vi "BlackBox232.vi"(5 "Input Command":string, 6 "VISA resource name":refnum<visa-resource-name>) -> (0 "error out 3":errorcluster, 1 "MonData":T2, 2 "MeasData":T1, 3 "Boolean":bool, 4 "String":string)   [LabVIEW 2010]
uses:
  <vilib>/Instr/_visa.llb/VISA Configure Serial Port (Instr).vi
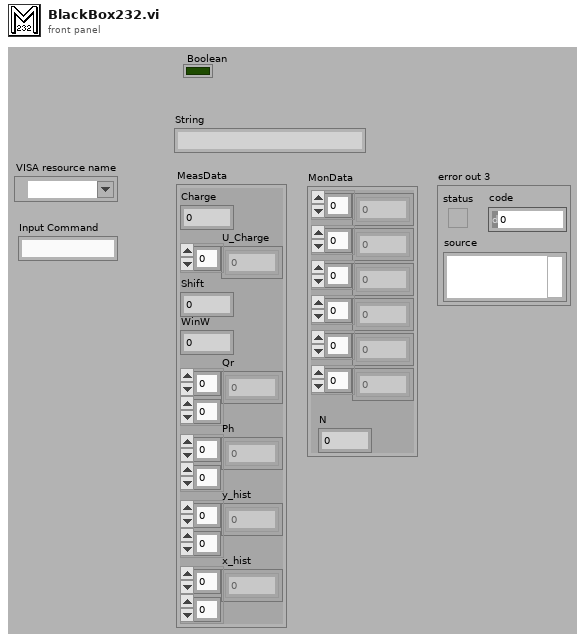
[diagram p1: front panel]
types:
  T1 = cluster{"Charge":i32, "U_Charge":i32[], "Shift":i32, "WinW":i32, "Qr":i32[][], "Ph":i32[][], "y_hist":i32[][], "x_hist":i32[][]}
  T2 = cluster{u16[], u16[], u16[], u16[], u16[], u16[], "N":i32}
  T3 = cluster{"Charge":i32, " U_Charge ":i32[], "Shift":i32, "WinW":i32, "Qr":i32[][], "Ph":i32[][], "y_hist":i32[][], "x_hist":i32[][]}
  T4 = cluster{u16[], u16[], u16[], u16[], u16[], u16[], dbl}
  T5 = cluster{u16[], u16[], u16[], u16[], u16[], u16[], "N":dbl}
  T6 = cluster{u16[], u16[], u16[], u16[], u16[], u16[], "Numeric":dbl}
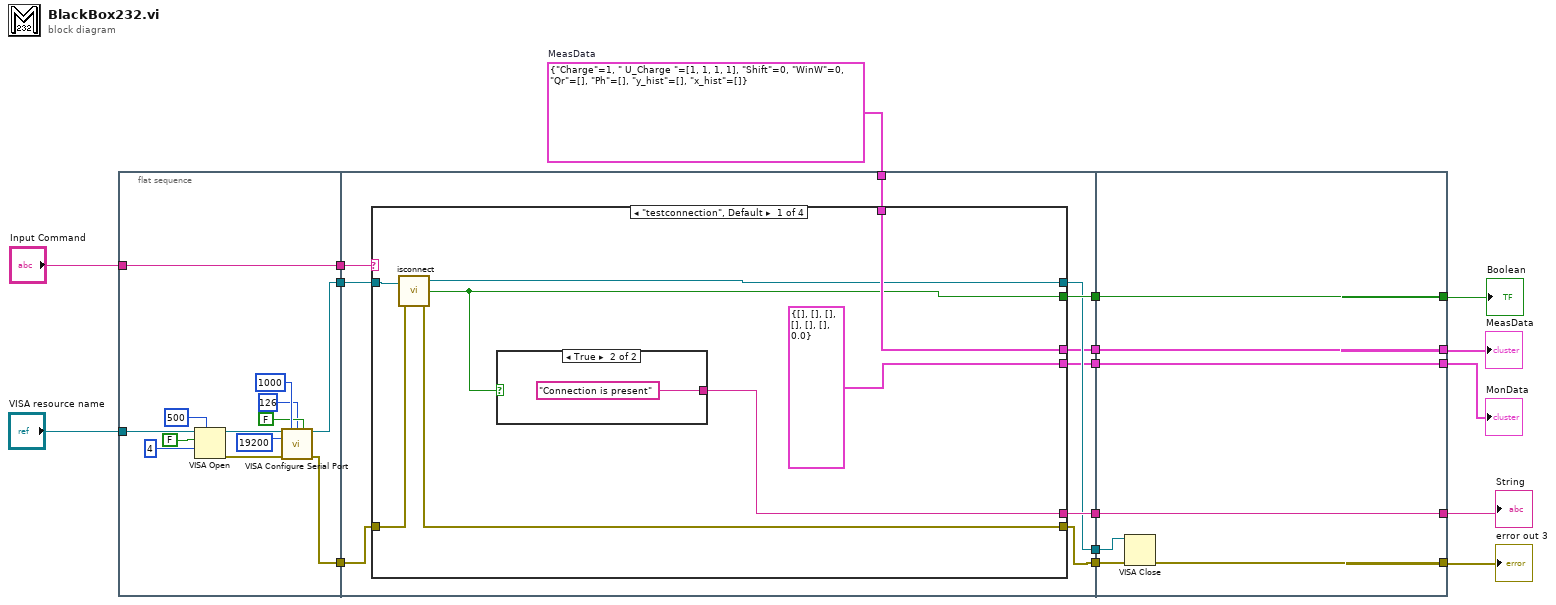
[diagram p0: block diagram]
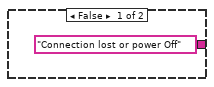
[diagram p2: hidden frame]
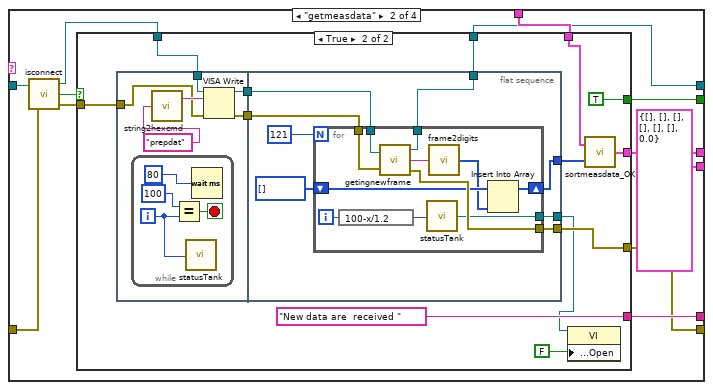
[diagram p3: hidden frame]
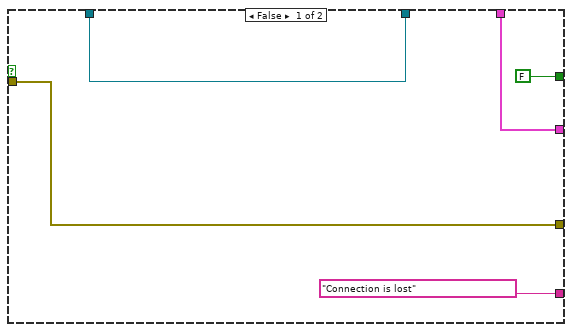
[diagram p4: hidden frame]
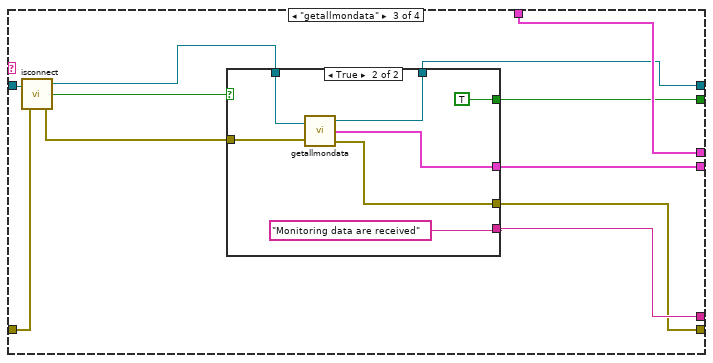
[diagram p5: hidden frame]
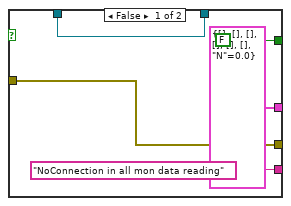
[diagram p6: hidden frame]
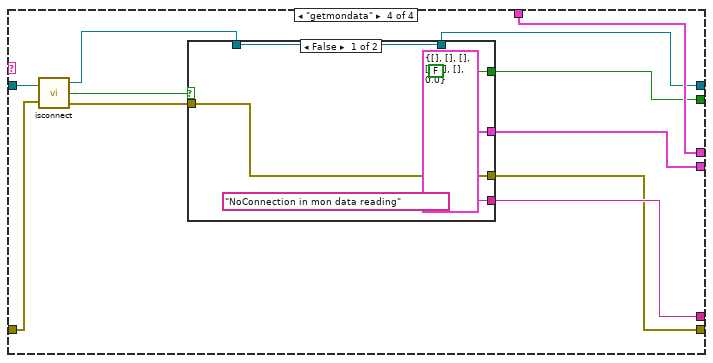
[diagram p7: hidden frame]
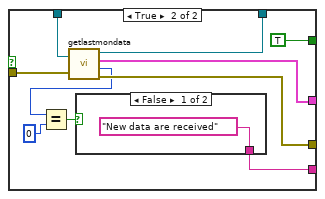
[diagram p8: hidden frame]
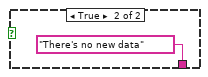
[diagram p9: hidden frame]
diagram:
  w3 = T3 {"Charge"=1, " U_Charge "=[1, 1, 1, 1], "Shift"=0, "WinW"=0, "Qr"=[], "Ph"=[], "y_hist"=[], "x_hist"=[]}  # MeasData
  n1 = flat-sequence {
    tunnel: [w18] -> w17
    tunnel: [w21] -> w16
    tunnel: [w20] -> w15
    tunnel: "VISA resource name" -> [w19]
    tunnel: "Input Command" -> [w18]
    tunnel: w17 -> [w40]
    tunnel: w16 -> [w39]
    tunnel: w15 -> [w38]
    tunnel: [w35] -> w14
    tunnel: [w33] -> w13
    tunnel: [w37] -> w12
    tunnel: w3 -> [w36]
    tunnel: [w34] -> w11
    tunnel: [w32] -> w10
    tunnel: [w31] -> w9
    tunnel: w14 -> [w167]
    tunnel: w13 -> [w166]
    tunnel: [w165] -> w2
    tunnel: w12 -> [w164]
    tunnel: [w164] -> w1
    tunnel: w11 -> [w163]
    tunnel: [w163] -> w4
    tunnel: [w162] -> w5
    tunnel: w10 -> [w162]
    tunnel: [w161] -> w6
    tunnel: w9 -> [w161]
    frame #0 {
      n2 = VISA Open(timeout (0)=u32 500 ("VISA Open timeout (0)"), duplicate session (F)=FALSE, access mode=u32 4, VISA resource name=w19) -> (VISA resource name=w22:refnum<visa-resource-name>, error out=w28:errorcluster)  [unwired: 1 in]
      n3 = call-poly "VISA Configure Serial Port"("VISA resource name"=w22, "timeout (10sec)"=u32 1000, "termination char\n(0xA = '\\n' = LF)"=u8 126 ("termination char\n(0xA = '\\n' = LF)"), "Enable Termination\nChar (T)"=FALSE ("Enable Termination\nChar (T)"), "baud rate (9600)"=u32 19200, "error in (no error)"=w28) -> ("VISA resource name out"=w21:refnum<visa-resource-name>, "error out"=w20:errorcluster)  [unwired: 8 in]
    }
    frame #1 {
      n4 = case shown="\"testconnection\", Default" w40 {
        tunnel: w39 -> [w46 w57 w120 w142]
        tunnel: w38 -> [w48 w58 w119 w136]
        tunnel: [w43 w62 w117 w138] -> w37
        tunnel: w36 -> [w47 w60 w118 w143]
        tunnel: [w47 w59 w118 w143] -> w32
        tunnel: [w45 w52 w112 w135] -> w35
        tunnel: [w42 w61 w115 w137] -> w34
        tunnel: [w44 w54 w110 w139] -> w33
        tunnel: [T4 {[], [], [], [], [], [], 0.0} ("output cluster") T4 {[], [], [], [], [], [], 0.0} ("output cluster") w114 w133] -> w31
        frame "testconnection", Default {
          n5 = call "isconnect.vi"("duplicate VISA resource name"=w46, "error in"=w48) -> ("dup VISA resource name"=w44:refnum<visa-resource-name>, "Boolean"=w43:bool, "error out"=w45:errorcluster)
          n6 = case shown="True" w43 {
            tunnel: ["Connection lost or power Off" "Connection is present"] -> w42
            frame False {
            }
            frame True {
            }
          }
        }
        frame "getmeasdata" {
          n7 = call "isconnect.vi"("duplicate VISA resource name"=w57, "error in"=w58) -> ("dup VISA resource name"=w55:refnum<visa-resource-name>, "Boolean"=w56:bool, "error out"=w53:errorcluster)
          n8 = case shown="True" w56 {
            tunnel: [FALSE TRUE] -> w62
            tunnel: ["Connection is lost" "New data are  received "] -> w61
            tunnel: w60 -> [w65 w74]
            tunnel: [w65 w75] -> w59
            tunnel: w55 -> [w64 w77]
            tunnel: [w64 w78] -> w54
            tunnel: w53 -> [w63 w72]
            tunnel: [w63 w70] -> w52
            frame False {
            }
            frame True {
              n9 = flat-sequence {
                tunnel: w77 -> [w86]
                tunnel: [w85] -> w76
                tunnel: w72 -> [w82]
                tunnel: [w81] -> w71
                tunnel: [w98] -> w78
                tunnel: [w94] -> w73
                tunnel: w76 -> [w97]
                tunnel: w71 -> [w96]
                tunnel: [w95] -> w70
                tunnel: [w91] -> w69
                frame #0 {
                  n10 = while {
                    i -> [w87]
                    stop <- w90 stop-if-true
                    n11 = Equal?(x=100, y=w87) -> (x = y?=w90:bool)
                    n12 = call "statusTank.vi"("Value"=w87) -> ()  [unwired: 1 out]
                    n13 = Wait (ms)(milliseconds to wait=80) -> ()  [unwired: 1 out]
                  }
                  n14 = call "string2hexcmd.vi"("String comand"="prepdat") -> ("hex comand"=w83:string)  [unwired: 1 out]
                  n15 = VISA Write(VISA resource name=w86, write buffer=w83, error in (no error)=w82) -> (VISA resource name out=w85:refnum<visa-resource-name>, error out=w81:errorcluster)  [unwired: 1 out]
                }
                frame #1 {
                  n16 = for {
                    N: 121 -> [_]
                    tunnel: w97 -> [w108]
                    tunnel: [w107] -> w98
                    tunnel: w96 -> [w105]
                    tunnel: [w104] -> w95
                    shift-right: [w102] -> w94
                    shift-left: u16[] [] -> [w103]
                    tunnel: [w99] -> w91
                    i -> [w109]
                    n17 = expression code="100-x/1.2"(w109) -> (w100:i32)
                    n18 = call "getingnewframe.vi"("dup VISA resource name 2"=w108, "error in (no error)"=w105) -> ("dup VISA resource name"=w107:refnum<visa-resource-name>, "data from COM Port"=w106:string, "error out"=w104:errorcluster)
                    n19 = call "statusTank.vi"("Value"=w100) -> ("vi reference"=w99:refnum<vi>)
                    n20 = call "frame2digits.vi"("data from COM Port"=w106) -> ("Digits"=w101:u16[])
                    n21 = Insert Into Array(array=w103, new element=w101) -> (w102:u16[])  [unwired: 1 in]
                  }
                }
              }
              n22 = property class="VI"(reference=w69, "Front Panel Window:Open"=FALSE) -> ()  [unwired: 1 in, 2 out]
              n23 = call "sortmeasdata_OK.vi"("Array"=w73, "MeasData 2"=w74) -> ("output cluster"=w75:T1)
            }
          }
        }
        frame "getallmondata" {
          n24 = call "isconnect.vi"("duplicate VISA resource name"=w120, "error in"=w119) -> ("dup VISA resource name"=w111:refnum<visa-resource-name>, "Boolean"=w116:bool, "error out"=w113:errorcluster)
          n25 = case shown="True" w116 {
            tunnel: [FALSE TRUE] -> w117
            tunnel: ["NoConnection in all mon data reading" "Monitoring data are received"] -> w115
            tunnel: [T5 {[], [], [], [], [], [], "N"=0.0} ("output cluster") w128] -> w114
            tunnel: w113 -> [w123 w130]
            tunnel: [w123 w129] -> w112
            tunnel: w111 -> [w121 w127]
            tunnel: [w121 w126] -> w110
            frame False {
            }
            frame True {
              n26 = call "getallmondata.vi"("duplicate VISA resource name"=w127, "error out 2"=w130) -> ("duplicate VISA resource name 2"=w126:refnum<visa-resource-name>, "output cluster"=w128:T2, "error out"=w129:errorcluster)
            }
          }
        }
        frame "getmondata" {
          n27 = call "isconnect.vi"("duplicate VISA resource name"=w142, "error in"=w136) -> ("dup VISA resource name"=w140:refnum<visa-resource-name>, "Boolean"=w134:bool, "error out"=w141:errorcluster)
          n28 = case shown="False" w134 {
            tunnel: [FALSE TRUE] -> w138
            tunnel: ["NoConnection in mon data reading" w150] -> w137
            tunnel: w140 -> [w145 w155]
            tunnel: [w145 w157] -> w139
            tunnel: w141 -> [w146 w156]
            tunnel: [w146 w154] -> w135
            tunnel: [T6 {[], [], [], [], [], [], "Numeric"=0.0} ("output cluster") w149] -> w133
            frame False {
            }
            frame True {
              n29 = call "getlastmondata.vi"("duplicate VISA resource name"=w155, "error out 2"=w156) -> ("duplicate VISA resource name 2"=w157:refnum<visa-resource-name>, "output cluster"=w149:T6, "N"=w152:u16, "error out"=w154:errorcluster)
              n30 = Equal?(x=w152, y=0) -> (x = y?=w151:bool)
              n31 = case shown="False" w151 {
                tunnel: ["New data are received" "There's no new data"] -> w150
                frame False {
                }
                frame True {
                }
              }
            }
          }
        }
      }
    }
    frame #2 {
      n32 = VISA Close(VISA resource name=w166, error in (no error)=w167) -> (error out=w165:errorcluster)
    }
  }
  "MonData" <- w6
  "MeasData" <- w5
  "String" <- w4
  "error out 3" <- w2
  "Boolean" <- w1
